vi "XML-RPC Response Parser.vi"(8 "error in (no error)":errorcluster, 11 "XML-RPC Call":string="HTTP/1.1 200 OK\nConnection: close\nContent-Length: 5461\nContent-Type: text/xml\nDate: Tue, 17 Apr 2007 14:06:55 GMT\nServer: LabVIEW 8.20/XP\n\n<?xml version=\"1.0\" encoding=\"UTF-8\"?>\n<methodResponse>\n  <params>\n    <param>\n      <array>\n  <data>\r<value><double>0.000000</double></value>\r<value><double>1.175571</double></value>\r<value><double>1.902113</double></value>\r<value><double>1.902113</double></value>\r<value><double>1.175571</double></value>\r<value><double>0.000000</double></value>\r<value><double>-1.175571</double></value>\r<value><double>-1.902113</double></value>\r<value><double>-1.902113</double></value>\r<value><double>-1.175571</double></value>\r<value><double>0.000000</double></value>\r<value><double>1.175571</double></value>\r<value><double>1.902113</double></value>\r<value><double>1.902113</double></value>\r<value><double>1.175571</double></value>\r<value><double>0.000000</double></value>\r<value><double>-1.175571</double></value>\r<value><double>-1.902113</double></value>\r<value><double>-1.902113</double></value>\r<value><double>-1.175571</double></value>\r<value><double>0.000000</double></value>\r<value><double>1.175571</double></value>\r<value><double>1.902113</double></value>\r<value><double>1.902113</double></value>\r<value><double>1.175571</double></value>\r<value><double>0.000000</double></value>\r<value><double>-1.175571</double></value>\r<value><double>-1.902113</double></value>\r<value><double>-1.902113</double></value>\r<value><double>-1.175571</double></value>\r<value><double>0.000000</double></value>\r<value><double>1.175571</double></value>\r<value><double>1.902113</double></value>\r<value><double>1.902113</double></value>\r<value><double>1.175571</double></value>\r<value><double>0.000000</double></value>\r<value><double>-1.175571</double></value>\r<value><double>-1.902113</double></value>\r<value><double>-1.902113</double></value>\r<value><double>-1.175571</double></value>\r<value><double>0.000000</double></value>\r<value><double>1.175571</double></value>\r<value><double>1.902113</double></value>\r<value><double>1.902113</double></value>\r<value><double>1.175571</double></value>\r<value><double>0.000000</double></value>\r<value><double>-1.175571</double></value>\r<value><double>-1.902113</double></value>\r<value><double>-1.902113</double></value>\r<value><double>-1.175571</double></value>\r<value><double>0.000000</double></value>\r<value><double>1.175571</double></value>\r<value><double>1.902113</double></value>\r<value><double>1.902113</double></value>\r<value><double>1.175571</double></value>\r<value><double>0.000000</double></value>\r<value><double>-1.175571</double></value>\r<value><double>-1.902113</double></value>\r<value><double>-1.902113</double></value>\r<value><double>-1.175571</double></value>\r<value><double>0.000000</double></value>\r<value><double>1.175571</double></value>\r<value><double>1.902113</double></value>\r<value><double>1.902113</double></value>\r<value><double>1.175571</double></value>\r<value><double>0.000000</double></value>\r<value><double>-1.175571</double></value>\r<value><double>-1.902113</double></value>\r<value><double>-1.902113</double></value>\r<value><double>-1.175571</double></value>\r<value><double>0.000000</double></value>\r<value><double>1.175571</double></value>\r<value><double>1.902113</double></value>\r<value><double>1.902113</double></value>\r<value><double>1.175571</double></value>\r<value><double>0.000000</double></value>\r<value><double>-1.175571</double></value>\r<value><double>-1.902113</double></value>\r<value><double>-1.902113</double></value>\r<value><double>-1.175571</double></value>\r<value><double>0.000000</double></value>\r<value><double>1.175571</double></value>\r<value><double>1.902113</double></value>\r<value><double>1.902113</double></value>\r<value><double>1.175571</double></value>\r<value><double>0.000000</double></value>\r<value><double>-1.175571</double></value>\r<value><double>-1.902113</double></value>\r<value><double>-1.902113</double></value>\r<value><double>-1.175571</double></value>\r<value><double>0.000000</double></value>\r<value><double>1.175571</double></value>\r<value><double>1.902113</double></value>\r<value><double>1.902113</double></value>\r<value><double>1.175571</double></value>\r<value><double>0.000000</double></value>\r<value><double>-1.175571</double></value>\r<value><double>-1.902113</double></value>\r<value><double>-1.902113</double></value>\r<value><double>-1.175571</double></value>\r<value><double>0.000000</double></value>\r<value><double>1.175571</double></value>\r<value><double>1.902113</double></value>\r<value><double>1.902113</double></value>\r<value><double>1.175571</double></value>\r<value><double>0.000000</double></value>\r<value><double>-1.175571</double></value>\r<value><double>-1.902113</double></value>\r<value><double>-1.902113</double></value>\r<value><double>-1.175571</double></value>\r<value><double>0.000000</double></value>\r<value><double>1.175571</double></value>\r<value><double>1.902113</double></value>\r<value><double>1.902113</double></value>\r<value><double>1.175571</double></value>\r<value><double>0.000000</double></value>\r<value><double>-1.175571</double></value>\r<value><double>-1.902113</double></value>\r<value><double>-1.902113</double></value>\r<value><double>-1.175571</double></value>\r<value><double>0.000000</double></value>\r<value><double>1.175571</double></value>\r<value><double>1.902113</double></value>\r<value><double>1.902113</double></value>\r<value><double>1.175571</double></value>\r<value><double>0.000000</double></value>\r<value><double>-1.175571</double></value>\r<value><double>-1.902113</double></value>\n  </data>\n</array>\n    </param>\n  </params>\n</methodResponse>") -> (0 "error out":errorcluster, 3 "Parameter":string)   [LabVIEW 2009]
doc: "This VI parses out and returns the response from an XML-RPC call"
panel:
  in  "XML-RPC Validation for  Method Call":string="<\\?xml version=\"1.0\".*\\?>[\\s\\n\\r\\t]*<methodResponse>[\\s\\n\\r\\t]*.*</methodResponse>"
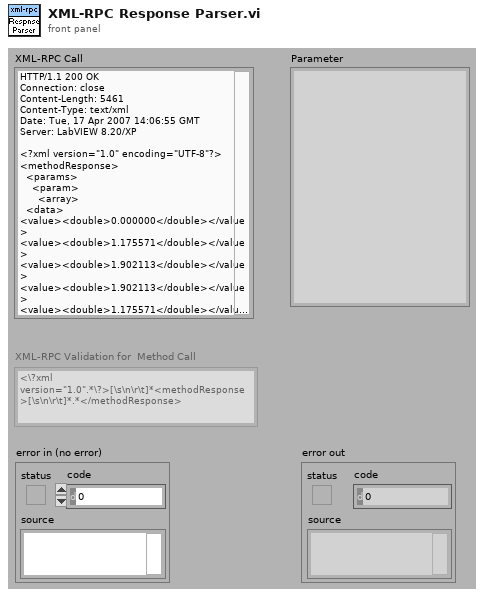
[diagram p1: front panel]
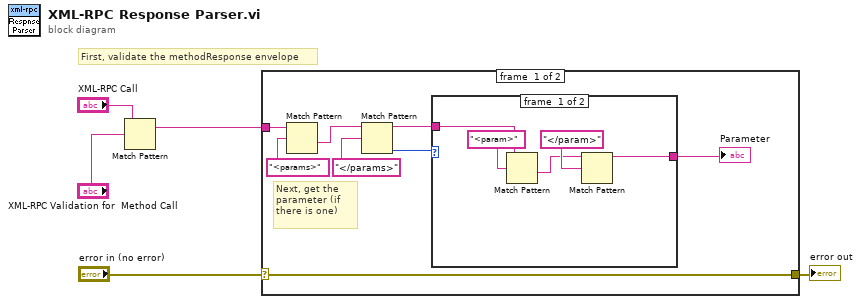
[diagram p0: block diagram]
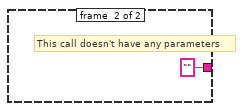
[diagram p2: hidden frame]
diagram:
  # "First, validate the methodResponse envelope"
  n1 = Match Pattern(string="XML-RPC Call", regular expression="XML-RPC Validation for  Method Call") -> (match substring=w2:string)  [unwired: 1 in, 3 out]
  n2 = case shown="No Error" "error in (no error)" {
    selector: "error in (no error)" -> [w13 w20]
    tunnel: [w13 w20] -> w3
    tunnel: w2 -> [w10 _]
    frame #0 {
      # "Next, get the parameter (if there is one)"
      n3 = Match Pattern(string=w10, regular expression="<params>") -> (after substring=w12:string)  [unwired: 1 in, 3 out]
      n4 = Match Pattern(string=w12, regular expression="</params>") -> (before substring=w7:string, offset past match=w8:i32)  [unwired: 1 in, 2 out]
      n5 = case shown="0, Default" w8 {
        tunnel: w7 -> [w18 _]
        tunnel: [w14 "" ("XML-RPC Call")] -> w6
        frame #0 {
          n6 = Match Pattern(string=w18, regular expression="<param>") -> (after substring=w16:string)  [unwired: 1 in, 3 out]
          n7 = Match Pattern(string=w16, regular expression="</param>") -> (before substring=w14:string)  [unwired: 1 in, 3 out]
        }
        frame #1 {
          # "This call doesn't have any parameters"
        }
      }
      "Parameter" <- w6
    }
    frame #1 {
    }
  }
  "error out" <- w3
